vi "Initialize.vi"(8 "error in":errorcluster, 10 "parameters":variant, 11 "cRIO in":refnum<class "PLTarget cRIO.lvclass">) -> (0 "error out":errorcluster, 2 "summary":T2[](array[typedef]), 3 "data value reference":T1)   [LabVIEW 2013, in "PLTarget cRIO.lvclass"]
doc: "This Vi initializes the data of a node its default state.\nThe object is not created inside of this ViI, beacuase it is created from a File depending on user selection."
uses:
  PLTarget cRIO.lvclass
  <vilib>/CEF_TreeControl/Node/Summary.ctl
  <vilib>/CEF_TreeControl/Node/NodeRef.ctl
  <vilib>/CEF_TreeControl/Node/NISE_CEF_Node.lvclass
  PLTarget cRIO.lvclass/PLTarget cRIO.ctl
  <vilib>/NI/Tag Bus Module Framework/root configuration/Target Types.ctl
  Framework Configuration Classes/target configuration/PL_Target Configuration.lvclass/PL_Target Configuration.ctl
  Configuration Editor/Classes/Targets/Targets.lvclass
  <vilib>/NI/Tag Bus Module Framework/root configuration/set metadata property.vi
  <vilib>/NI/Tag Bus Module Framework/root configuration/TBM configuration.lvclass
  Framework Configuration Classes/target configuration/PL_Target Configuration.lvclass
  Configuration Editor/Classes/TBM Configuration Node/TBM Configuration Node.lvclass
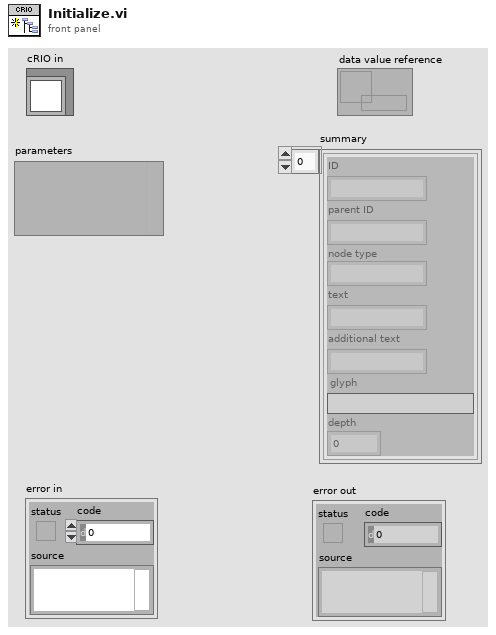
[diagram p1: front panel]
types:
  T1 = typedef "NISE_CEF_Node.lvclass/NodeRef.ctl" = refnum<data-value>
  T2 = typedef "NISE_CEF_Node.lvclass/Summary.ctl" = cluster{"ID":string, "parent ID":string, "node type":string, "text":string, "additional text":string, "glyph":string, "depth":i32}
  T3 = typedef "TBM configuration.lvclass/Target Types.ctl" = enum16{"Windows", "Mac", "Linux", "Linux RT ARM", "VxWorks", "Pharlap", "Other", "Linux RT x64"}
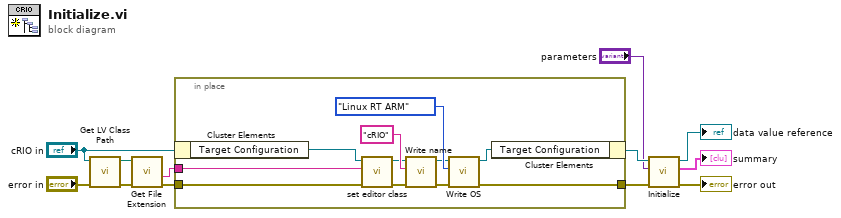
[diagram p0: block diagram]
diagram:
  n1 = call <vilib>:"Get LV Class Path.vi"("error in (no error)"="error in", "object"="cRIO in") -> ("error out"=w6:errorcluster, "class path"=w5:path)  [unwired: 8 in]
  n2 = call <vilib>:"Get File Extension.vi"("error in (no error)"=w6, "file"=w5) -> ("error out"=w2:errorcluster, "filename without extension"=w1:string)  [unwired: 6 in, 2 out]
  n3 = in-place {
    in-place-border: [w21] -> w9
    in-place-border: w2 -> [w22]
    in-place-border: w1 -> [w13]
    n4 = in-place-cluster #1("cRIO in") -> ("Target Configuration"=w15:refnum<class "PL_Target Configuration.lvclass">)
    n5 = call "set editor class.vi"("error in"=w22, "editor class"=w13, "configuration in"=w15) -> ("error out"=w16:errorcluster, "configuration out"=w14:refnum<class "PL_Target Configuration.lvclass">)  [unwired: 7 in]
    n6 = call "Write name.vi"("error in"=w16, "name"="cRIO", "PL_Local Target Configuration in"=w14) -> ("error out"=w18:errorcluster, "PL_Local Target Configuration out"=w19:refnum<class "PL_Target Configuration.lvclass">)  [unwired: 7 in]
    n7 = call "Write OS.vi"("error in"=w18, "Target Types"=Target_Types."Linux RT ARM" ("OS"), "PL_Target Configuration in"=w19) -> ("error out"=w21:errorcluster, "PL_Target Configuration out"=w17:refnum<class "PL_Target Configuration.lvclass">)  [unwired: 7 in]
    n8 = in-place-cluster #1("Target Configuration"=w17) -> (w8:refnum<class "PLTarget cRIO.lvclass">)
  }
  n9 = call-parent "Initialize.vi"("error in"=w9, "parameters"="parameters", "node in"=w8) -> ("error out"=→"error out":errorcluster, "summary"=→"summary":T2[], "data value reference"=→"data value reference":T1)  [unwired: 6 in]
